vi "写配置设置文件.vi"() -> ()   [LabVIEW 2010]
doc: "Illustrates how to create and write a configuration settings file.\n\nInstructions:\nEnter values in the controls on the front panel then click on the Run Arrow.\nTo read the file, run Read Configuration Settings File.vi located in the file\\config.llb."
uses:
  <vilib>/Utility/config.llb/Write Key (Path).vi
  <vilib>/Utility/config.llb/Write Key (Double).vi
  <vilib>/Utility/config.llb/NI_LVConfig.lvlib
panel:
  in  "min":dbl=80.0 format="%.2f"
  in  "max":dbl=100.0 format="%.2f"
  in  "Path Value":path=path "C:/My Path Name"
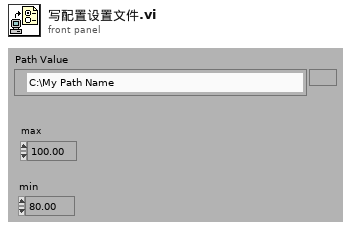
[diagram p1: front panel]
types:
  T1 = typedef "NI_LVConfig.lvlib/Config Data RefNum.ctl" = refnum<k1>
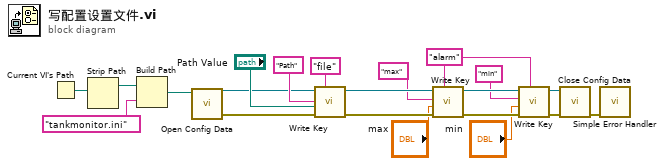
[diagram p0: block diagram]
diagram:
  w10 = "alarm"
  n1 = Current VI's Path() -> (path=w5:path)
  n2 = Strip Path(path=w5) -> (stripped path=w6:path)  [unwired: 1 out]
  n3 = Build Path(base path=w6, name or relative path="tankmonitor.ini") -> (appended path=w3:path)
  n4 = call <vilib>:"Open Config Data.vi"("configuration file path"=w3) -> ("error out"=w1:errorcluster, "refnum"=w2:T1)  [unwired: 8 in, 1 out]
  n5 = call-poly <vilib>:"Write Key.vi"("section"="file", "error in (no error)"=w1, "value"="Path Value", "key"="Path" ("Key 3"), "refnum"=w2) -> ("error out"=w18:errorcluster, "refnum out"=w21:T1)  [unwired: 4 in, 1 out]
  n6 = call-poly <vilib>:"Write Key.vi"("section"=w10, "error in (no error)"=w18, "value"="max", "key"="max" ("Key 4"), "refnum"=w21) -> ("error out"=w17:errorcluster, "refnum out"=w20:T1)  [unwired: 4 in, 1 out]
  n7 = call-poly <vilib>:"Write Key.vi"("section"=w10, "error in (no error)"=w17, "value"="min", "key"="min" ("Key 5"), "refnum"=w20) -> ("error out"=w16:errorcluster, "refnum out"=w19:T1)  [unwired: 4 in, 1 out]
  n8 = call <vilib>:"Close Config Data.vi"("error in (no error)"=w16, "refnum"=w19) -> ("error out"=w12:errorcluster)  [unwired: 8 in, 1 out]
  n9 = call <vilib>:"Simple Error Handler.vi"("error in (no error)"=w12) -> ()  [unwired: 4 in, 5 out]
